vi "FPGA Read FIFO - U8.vi"(6 "Timeout (ms)":u32=5000, 8 "error in (no error)":errorcluster, 9 "Number of Elements":u32, 10 "FIFO":T1, 11 "FPGA Session In":refnum<class "Firmware Independent PID Interface.lvclass">) -> (0 "error out":errorcluster, 1 "Elements Remaining":u32, 2 "Data":u8[](array[numeric]), 3 "FPGA Session Out":refnum<class "Firmware Independent PID Interface.lvclass">)   [LabVIEW 2010, in "Firmware Independent PID Interface.lvclass"]
doc: "Reads from a FIFO of unsigned 8-bit integers."
uses:
  Firmware Independent PID Interface.lvclass
  TypeDefs/TargetToHostFifoU8.ctl
  <vilib>/rvi/DataTransferAndStorage/Container/Common/niFpgaDataTypeControl.ctl
  <userlib>/_FPGA Interface Advanced Tools/FPGA Interface Base/FPGA Interface Base.lvclass/FPGA Interface Base.ctl
  <vilib>/Utility/error.llb/Error Cluster From Error Code.vi
  <userlib>/_FPGA Interface Advanced Tools/FPGA Interface Base/Accessors/FPGA Read Session.vi
  <userlib>/_FPGA Interface Advanced Tools/FPGA Interface Wrapper/FPGA Interface Wrapper.lvlib
  <userlib>/_FPGA Interface Advanced Tools/FPGA Interface Base/FPGA Interface Base.lvclass
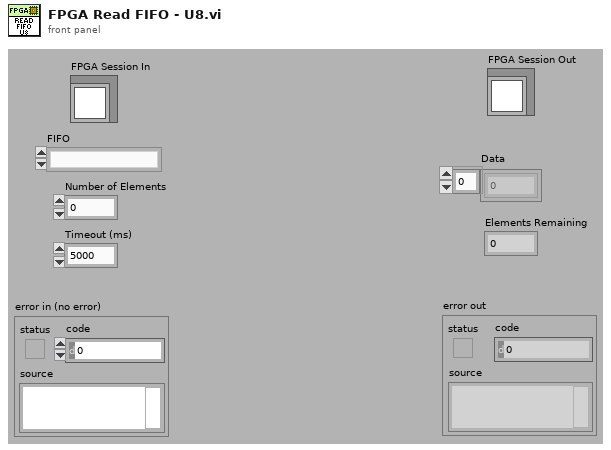
[diagram p1: front panel]
types:
  T1 = typedef "Firmware Independent PID Interface.lvclass/TargetToHostFifoU8.ctl" = enum16{""}
  T2 = typedef "niFpgaDataTypeControl.ctl" = enum32{"Boolean", "I8", "I16", "I32", "I64", "U8", "U16", "U32", "U64", "FXP", "CustomControl"}
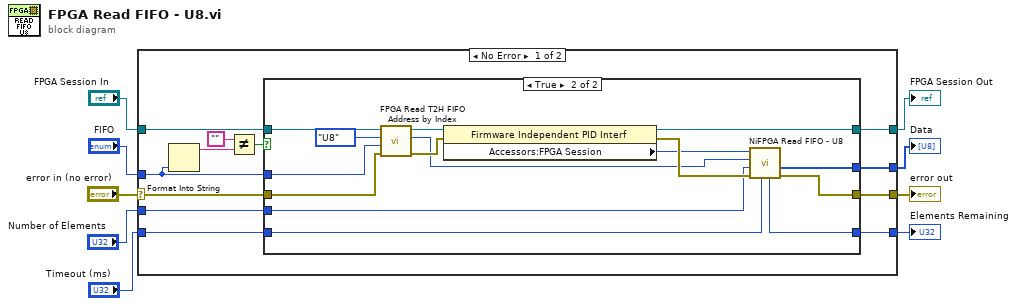
[diagram p0: block diagram]
diagram:
  n1 = case shown="No Error" "error in (no error)" {
    selector: "error in (no error)" -> [w10 w40]
    tunnel: [w12 w40] -> w1
    tunnel: [w14 w39] -> w4
    tunnel: [w13 _] -> w3
    tunnel: "FPGA Session In" -> [w19 w39]
    tunnel: "FIFO" -> [w17 _]
    tunnel: [w11 _] -> w2
    tunnel: "Number of Elements" -> [w16 _]
    tunnel: "Timeout (ms)" -> [w15 _]
    frame No Error {
      n2 = Format Into String(w17) -> (resulting string=w21:string)  [unwired: 3 in, 1 out]
      n3 = Not Equal?(x="", y=w21) -> (x != y?=w18:bool)
      n4 = case shown="True" w18 {
        tunnel: [w22 w34] -> w12
        tunnel: [w23 w35] -> w14
        tunnel: [_ w38] -> w13
        tunnel: w19 -> [w23 w33]
        tunnel: w17 -> [_ w31]
        tunnel: [_ w27] -> w11
        tunnel: w16 -> [_ w26]
        tunnel: w15 -> [_ w25]
        tunnel: w10 -> [w22 w24]
        frame False {
        }
        frame True {
          n5 = call <userlib>:"FPGA Read T2H FIFO Address by Index.vi"("error in (no error)"=w24, "index"=w31, "Data Type"=niFpgaDataTypeControl."U8", "FPGA Interface Base in"=w33) -> ("error out"=w29:errorcluster, "Address"=w28:u32, "FPGA Interface Base out"=w32:refnum<class "Firmware Independent PID Interface.lvclass">)  [unwired: 4 in, 1 out]
          n6 = property class="Firmware Independent PID Interf"(reference=w32, error in=w29) -> (reference out=w35:refnum<class "Firmware Independent PID Interface.lvclass">, error out=w37:errorcluster, "Accessors:FPGA Session"=w36:u32)
          n7 = call <userlib>:"NiFPGA Read FIFO - U8.vi"("Timeout"=w25, "error in (no error)"=w37, "Number of Elements"=w26, "FIFO"=w28, "Session"=w36) -> ("error out"=w34:errorcluster, "Data"=w38:u8[], "Elements Remaining"=w27:u32)  [unwired: 3 in, 1 out]
        }
      }
    }
    frame Error {
    }
  }
  "error out" <- w1
  "FPGA Session Out" <- w4
  "Data" <- w3
  "Elements Remaining" <- w2
